vi "ResultTable.vi"(8 "error in (no error)":errorcluster, 10 "AllData":T1 {"FlukeData"."DataAnalysisArray"."TimeStamp" format="%^<%.3X\n%x>T"; "FlukeData"."ModelDataArray"."FREQUENCY" format="%#_6f"; "FlukeData"."ModelDataArray"."TimeStamp" format="%^<%.3X\n%x>T"; "FlukeData"."PMUDataArray"."FREQUENCY" format="%#_6f"; "FlukeData"."PMUDataArray"."TimeStamp" format="%^<%.3X\n%x>T"; "NISTData"."DataAnlysisArray"."TimeStamp" format="%^<%.3X\n%x>T"; "NISTData"."DUTDataArray"."Time Stamp" format="%^<%.3X\n%x>T"; "NISTData"."NIDataArray"."Time Stamp" format="%^<%.3X\n%x>T"}, 11 "TVEMePe":dbl[][](array[numeric])) -> (0 "error out":errorcluster, 3 "Results Table":string[][](table))   [LabVIEW 2014]
uses:
  typedefs/Alldata.ctl
  typedefs/NISTData.ctl
  typedefs/NIDataArray.ctl
  typedefs/NIData.ctl
  typedefs/PhasorRectangular.ctl
  typedefs/DUTData.ctl
  typedefs/NICalcAnalysis.ctl
  typedefs/CalcPhasorError.ctl
  typedefs/PlotDataArrays.ctl
  typedefs/PmuRawDataCluster.ctl
  typedefs/CalcAnalysis.ctl
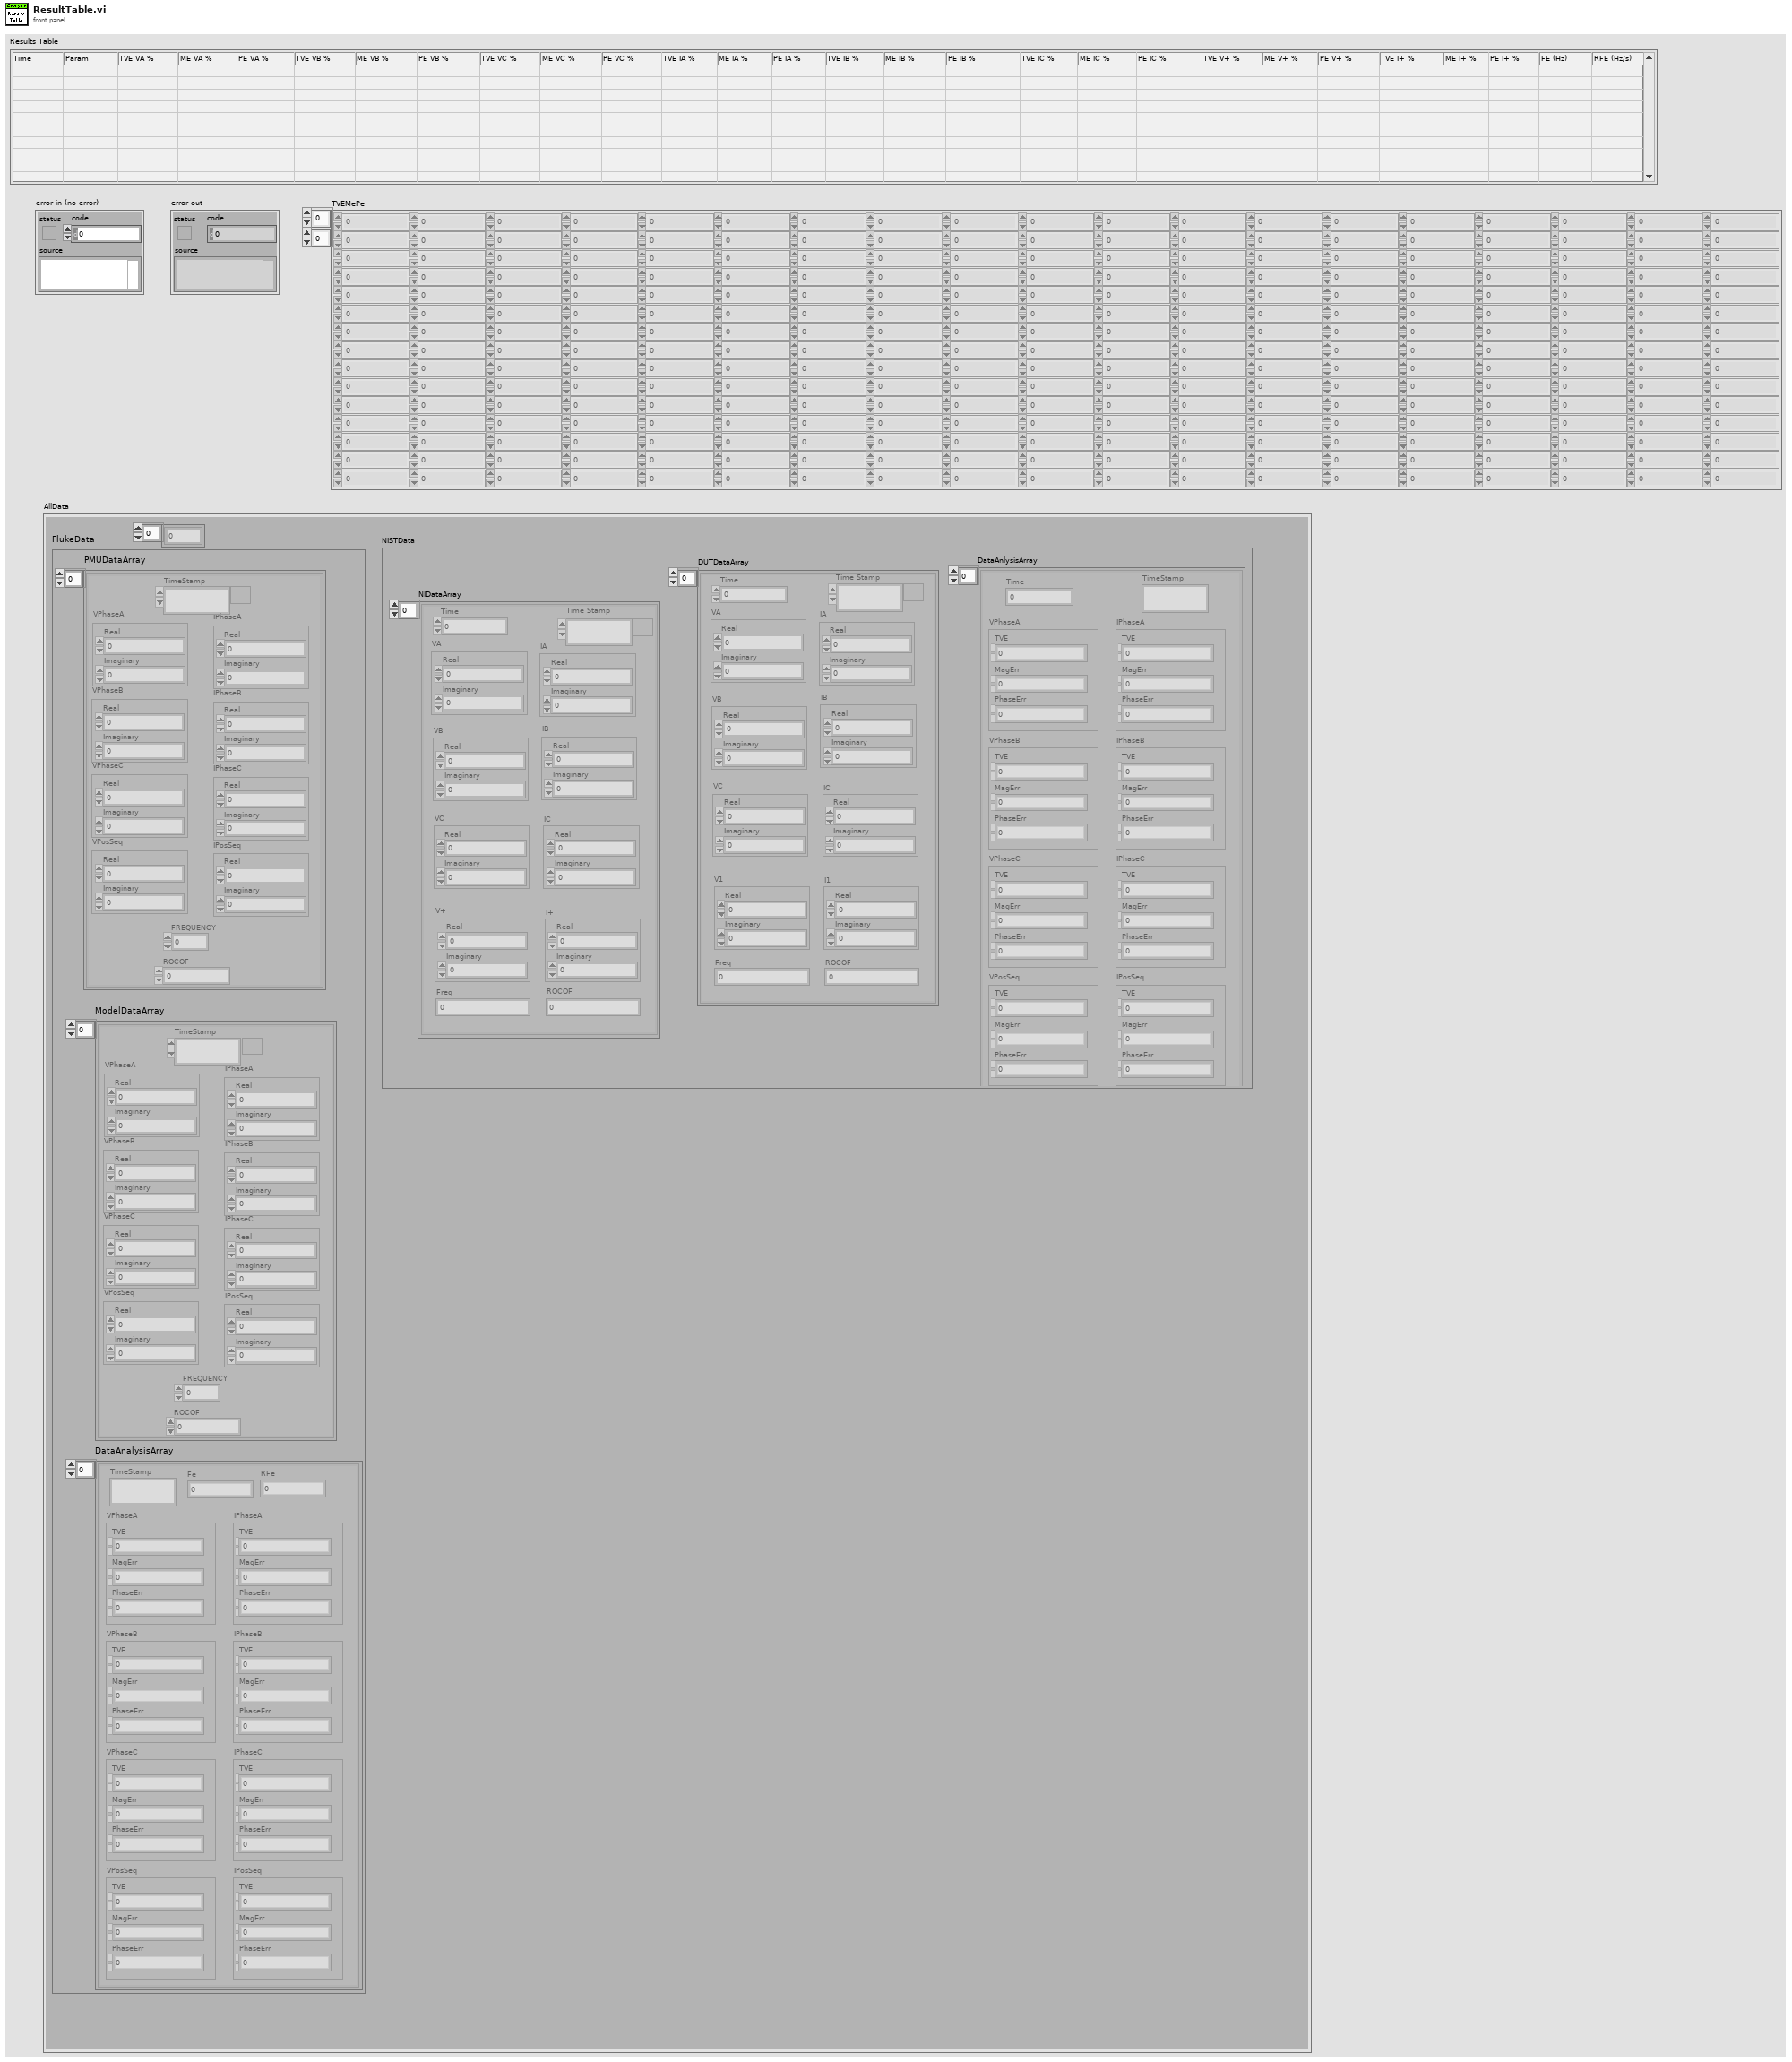
[diagram p1: front panel]
types:
  T1 = typedef "Alldata.ctl" = cluster{"NISTData":T2, "FlukeData":T9, "Params":dbl[]}
  T2 = typedef "NISTData.ctl" = cluster{"NIDataArray":T3, "DUTDataArray":T6[], "DataAnlysisArray":T7[]}
  T3 = typedef "NIDataArray.ctl" = T4[]
  T4 = typedef "NIData.ctl" = cluster{"Time":dbl, "VA":T5, "VB":T5, "VC":T5, "V+":T5, "IA":T5, "IB":T5, "IC":T5, "I+":T5, "Freq":dbl, "ROCOF":dbl, "Time Stamp":timestamp}
  T5 = typedef "PhasorRectangular.ctl" = cluster{"Real":dbl, "Imaginary":dbl}
  T6 = typedef "DUTData.ctl" = cluster{"Time":dbl, "VA":T5, "VB":T5, "VC":T5, "V1":T5, "IA":T5, "IB":T5, "IC":T5, "I1":T5, "Freq":dbl, "ROCOF":dbl, "Time Stamp":timestamp}
  T7 = typedef "NICalcAnalysis.ctl" = cluster{"Time":dbl, "VPhaseA":T8, "IPhaseA":T8, "VPhaseB":T8, "IPhaseB":T8, "VPhaseC":T8, "IPhaseC":T8, "VPosSeq":T8, "IPosSeq":T8, "Fe":dbl, "RFe":dbl, "TimeStamp":timestamp}
  T8 = typedef "CalcPhasorError.ctl" = cluster{"TVE":dbl, "MagErr":dbl, "PhaseErr":dbl}
  T9 = typedef "PlotDataArrays.ctl" = cluster{"PMUDataArray":T10[], "ModelDataArray":T10[], "DataAnalysisArray":T11[]}
  T10 = typedef "PmuRawDataCluster.ctl" = cluster{"TimeStamp":timestamp, "VPhaseA":T5, "VPhaseB":T5, "VPhaseC":T5, "VPosSeq":T5, "IPhaseA":T5, "IPhaseB":T5, "IPhaseC":T5, "IPosSeq":T5, "FREQUENCY":dbl, "ROCOF":sgl}
  T11 = typedef "CalcAnalysis.ctl" = cluster{"TimeStamp":timestamp, "VPhaseA":T8, "VPhaseB":T8, "VPhaseC":T8, "VPosSeq":T8, "IPhaseA":T8, "IPhaseB":T8, "IPhaseC":T8, "IPosSeq":T8, "Fe":dbl, "RFe":dbl}
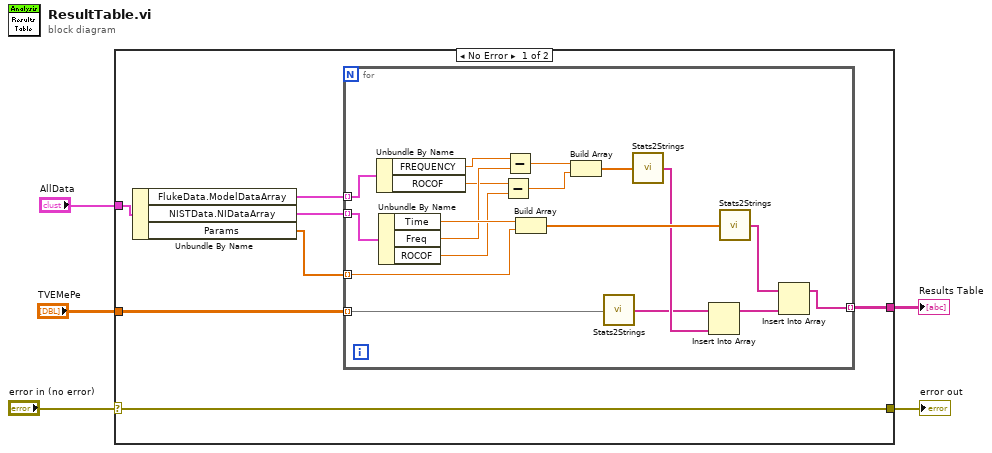
[diagram p0: block diagram]
diagram:
  n1 = case shown="No Error" "error in (no error)" {
    selector: "error in (no error)" -> [w11 w32]
    tunnel: [w11 w32] -> w4
    tunnel: "TVEMePe" -> [w12 _]
    tunnel: [w8 string[][] [] ("Strings")] -> w2
    tunnel: "AllData" -> [w10 _]
    frame No Error {
      n2 = Unbundle By Name(w10) -> ("FlukeData.ModelDataArray"=w7:T10[], "NISTData.NIDataArray"=w9:T3, "Params"=w6:dbl[])
      n3 = for {
        tunnel: w12 -> [w30] mode=indexing
        tunnel: w9 -> [w29] mode=indexing
        tunnel: [w26] -> w8 mode=indexing
        tunnel: w7 -> [w24] mode=indexing
        tunnel: w6 -> [w13] mode=indexing
        n4 = Unbundle By Name(w24) -> ("FREQUENCY"=w23:dbl, "ROCOF"=w21:sgl)
        n5 = Unbundle By Name(w29) -> ("Time"=w28:dbl, "Freq"=w22:dbl, "ROCOF"=w20:dbl)
        n6 = Subtract(x=w21, y=w20) -> (x-y=w18:dbl)
        n7 = Subtract(x=w23, y=w22) -> (x-y=w19:dbl)
        n8 = Build Array(w28, w13) -> (w27:dbl[])
        n9 = Build Array(w19, w18) -> (w17:dbl[])
        n10 = call "Stats2Strings.vi"("stats"=w30) -> ("Strings"=w15:string[])  [unwired: 8 in]
        n11 = call "Stats2Strings.vi"("stats"=w17) -> ("Strings"=w16:string[])  [unwired: 8 in]
        n12 = Insert Into Array(array=w15, new element=w16) -> (w14:string[])  [unwired: 1 in]
        n13 = call "Stats2Strings.vi"("stats"=w27) -> ("Strings"=w25:string[])  [unwired: 8 in]
        n14 = Insert Into Array(array=w25, new element=w14) -> (w26:string[])  [unwired: 1 in]
      }
    }
    frame Error {
    }
  }
  "Results Table" <- w2
  "error out" <- w4
